vi "solar_voy Export.vi"(6 "Suppress Errors? (T)":bool=TRUE, 8 "error in (no error)":errorcluster, 10 "COSMOS Root (\"\" = Use Default)":path, 11 "Voyager Refnum in":T1) -> (0 "error out":errorcluster, 3 "Voyager Refnum out":T1)   [LabVIEW 2018]
doc: "This exports all packets and interfaces to the root COSMOS directory. If the <b>COSMOS Root</b> is empty, this exports the definitions to the path specified in the Voyager reference."
uses:
  solar_voy_ctl Voyager Refnum.ctl
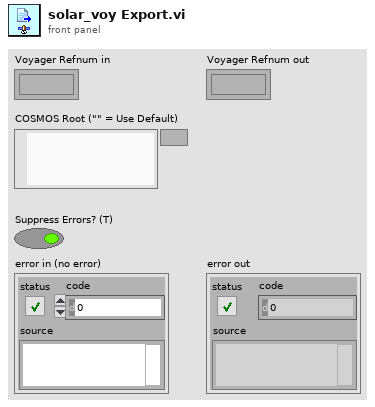
[diagram p1: front panel]
types:
  T1 = typedef "solar_voy_ctl Voyager Refnum.ctl" = refnum<k1>
  T2 = typedef "solar_voy_ctl Voyager.ctl" = cluster{"PACKETS":T3[], "COSMOS_Root":path, "CMD_HDR":T8, "TLM_HDR":T8, "TCPs":T9[], "VoyagerIDOffset":cluster{"VoyagerIDOffset":u16[], "Target Names":string[]}}
  T3 = typedef "solar_voy_def_ctl PACKET.ctl" = cluster{"PACKET_ID":T4, "ENDIAN":enum8{"BIG", "LITTLE"}, "DESC":string, "HZRD":bool, "ITEMS":T5[], "NoExport":bool, "last_time":timestamp, "last_count":u32, "last_data":string}
  T4 = typedef "solar_voy_def_ctl PACKET_ID.ctl" = cluster{"ID":u16, "CMD":enum8{"CMD", "TLM"}, "TARGET":string, "PACKET":string}
  T5 = typedef "solar_voy_def_ctl ITEM.ctl" = cluster{"NAME":string, "OFFSET":i32, "SIZE":i32, "TYPE":T6, "EACH_SIZE":i32, "LVTYPE":T7, "MIN":dbl, "MAX":dbl, "DEFAULT":string, "DESC":string, "ID":bool, "MODIFIERS":variant, "last_value":variant}
  T6 = typedef "solar_voy_def_ctl ITEM TYPE.ctl" = enum8{"BLOCK", "INT", "UINT", "FLOAT", "STRING"}
  T7 = typedef "solar_type Item Type.ctl" = enum16{"NULL", "UNKNOWN", "CLUSTER", "I8", "I16", "I32", "I64", "U8", "U16", "U32", "U64", "U8_ENUM", "U16_ENUM", "U32_ENUM", "SGL", "DBL", "BOOLEAN", "STRING", "PATH", "VISA", "TAG", "TIME", "I8_1D", "I16_1D", "I32_1D", "I64_1D", "U8_1D", "U16_1D", "U32_1D", "U64_1D", "U8_ENUM_1D", "U16_ENUM_1D", "U32_ENUM_1D", "SGL_1D", "DBL_1D", "BOOLEAN_1D", "STRING_1D", "PATH_1D", "VISA_1D", "TAG_1D", "TIME_1D", "I8_2D", "I16_2D", "I32_2D", "I64_2D", "U8_2D", "U16_2D", "U32_2D", "U64_2D", "U8_ENUM_2D", "U16_ENUM_2D", "U32_ENUM_2D", "SGL_2D", "DBL_2D", "BOOLEAN_2D", "STRING_2D", "PATH_2D", "VISA_2D", "TAG_2D", "TIME_2D"}
  T8 = typedef "solar_voy_def_ctl HDR.ctl" = cluster{"ITEMS":T5[], "LENGTH_NAME":string, "LENGTH_VALUE_OFFSET":i32, "ID_NAME":string, "ENDIAN":enum8{"BIG", "LITTLE"}, "GUID_NAME":string, "DEFAULT_TARGET":string, "DEFAULT_PACKET":string, "DEFAULT_ERROR":string}
  T9 = typedef "solar_voy_ctl TCP.ctl" = cluster{"Connected":bool, "Port":u16, "Listener":refnum<k5>, "ServerIP":string, "TCP":refnum<k5>, "Setup":T10, "VIRefnum":refnum<vi>, "TARGETS_CMD":string[], "TARGETS_TLM":string[]}
  T10 = typedef "solar_voy_ctl Port Setup.ctl" = enum8{"SERVER", "CLIENT", "SERVER_CMD", "SERVER_TLM"}
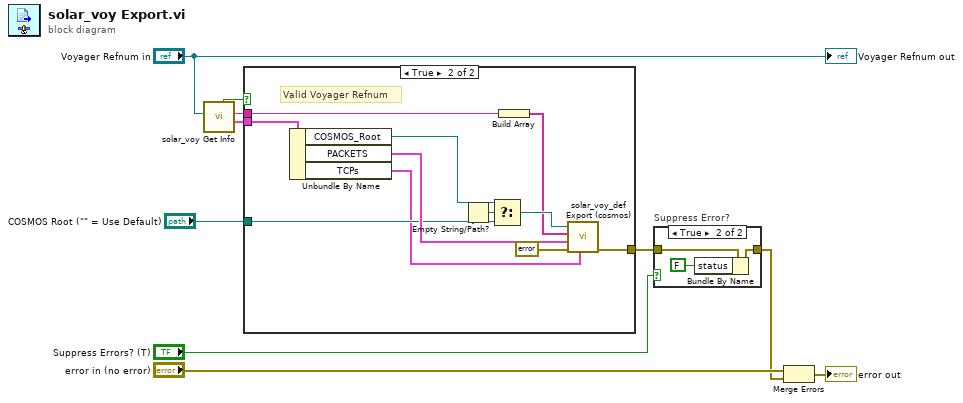
[diagram p0: block diagram]
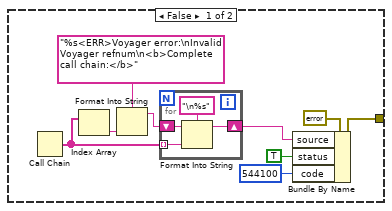
[diagram p2: hidden frame]
diagram:
  n1 = call "solar_voy Get Info.vi"("Voyager Refnum"="Voyager Refnum in") -> ("Voyager"=w3:T2, "Interface Name"=w2:string, "Valid Refnum?"=w4:bool)  [unwired: 8 in]
  n2 = case shown="True" w4 {
    tunnel: [w11 w32] -> w6
    tunnel: w3 -> [_ w34]
    tunnel: w2 -> [_ w31]
    tunnel: "COSMOS Root (\"\" = Use Default)" -> [_ w28]
    frame False {
      n3 = Call Chain() -> (call chain=w14:string[])
      n4 = Index Array(array=w14) -> (element=w16:string)  [unwired: 1 in]
      n5 = Format Into String(format string="%s<ERR>Voyager error:\nInvalid Voyager refnum\n<b>Complete call chain:</b>", w16) -> (resulting string=w15:string)  [unwired: 2 in, 1 out]
      n6 = for {
        tunnel: w14 -> [w23] mode=indexing
        shift-right: [w22] -> w13
        shift-left: w15 -> [w21]
        n7 = Format Into String(format string="\n%s", initial string=w21, w23) -> (resulting string=w22:string)  [unwired: 1 in, 1 out]
      }
      n8 = Bundle By Name(cluster=errorcluster {"status"=FALSE, "code"=0, "source"=""} ("error in (no error)"), "source"=w13, "status"=TRUE, "code"=544100 ("Code")) -> (w11:errorcluster)
    }
    frame True {
      # "Valid Voyager Refnum"
      n9 = Unbundle By Name(w34) -> ("COSMOS_Root"=w27:path, "PACKETS"=w30:T3[], "TCPs"=w25:T9[])
      n10 = Empty String/Path?(string/path=w28) -> (empty?=w29:bool)
      n11 = Select(t=w27, s=w29, f=w28) -> (s? t:f=w26:path)
      n12 = Build Array(w31) -> (w24:string[])
      n13 = call "solar_voy_def Export (cosmos).vi"("TCPs"=w25, "error in (no error)"=errorcluster {"status"=FALSE, "code"=0, "source"=""}, "ALL PACKETS"=w30, "Interface Names (\"\" = First Target)"=w24, "CosmosDir"=w26) -> ("error out"=w32:errorcluster)  [unwired: 5 in, 1 out]
    }
  }
  n14 = case "Suppress Error?" shown="True" "Suppress Errors? (T)" {
    tunnel: w6 -> [w35 w38]
    tunnel: [w35 w37] -> w8
    frame False {
    }
    frame True {
      n15 = Bundle By Name(cluster=w38, "status"=FALSE) -> (w37:errorcluster)
    }
  }
  n16 = Merge Errors("error in (no error)", w8) -> (→"error out":errorcluster)
  "Voyager Refnum out" <- "Voyager Refnum in"
